vi "stopReading.vi"(8 "error in (no error)":errorcluster, 10 "InternalCommandId.lvclass":refnum<class "InternalCommandId.lvclass">, 11 "ElectrometerController in":refnum<class "ElectrometerController.lvclass">) -> (0 "error out":errorcluster, 3 "ElectrometerController out":refnum<class "ElectrometerController.lvclass">)   [LabVIEW 2016, in "ElectrometerController.lvclass"]
uses:
  ElectrometerController.lvclass
  InternalCommandId/InternalCommandId.lvclass
  Electrometer/State/ElectrometerState.lvclass
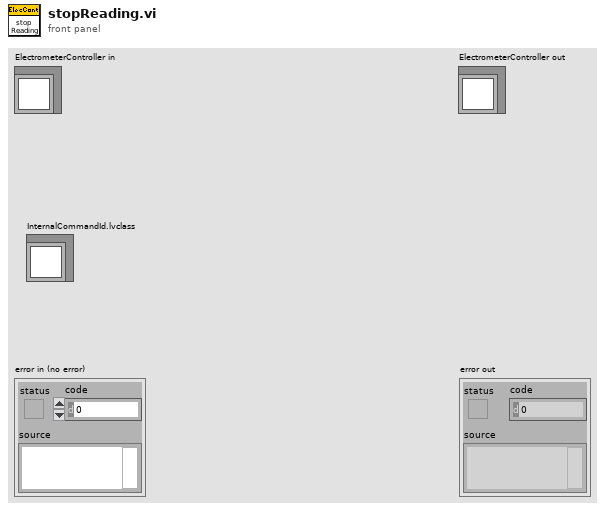
[diagram p1: front panel]
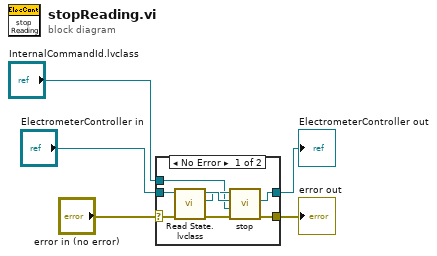
[diagram p0: block diagram]
diagram:
  n1 = case shown="No Error" "error in (no error)" {
    selector: "error in (no error)" -> [w9 w15]
    tunnel: [w8 w15] -> w4
    tunnel: [w10 w14] -> w2
    tunnel: "ElectrometerController in" -> [w13 w14]
    tunnel: "InternalCommandId.lvclass" -> [w6 _]
    frame No Error {
      n2 = call-dynamic "Read State.lvclass.vi"("error in (no error)"=w9, "ElectrometerController in"=w13) -> ("error out"=w7:errorcluster, "ElectrometerState"=w11:refnum<class "ElectrometerState.lvclass">, "ElectrometerController out"=w12:refnum<class "ElectrometerController.lvclass">)  [unwired: 7 in]
      n3 = call-dynamic "stop.vi"("error in (no error)"=w7, "InternalCommandId.lvclass"=w6, "ElectrometerController int"=w12, "State in"=w11) -> ("error out"=w8:errorcluster, "ElectrometerController out"=w10:refnum<class "ElectrometerController.lvclass">)  [unwired: 5 in, 1 out]
    }
    frame Error {
    }
  }
  "error out" <- w4
  "ElectrometerController out" <- w2
